vi "EnableDisable RTM.vi"(8 "error in (no error)":errorcluster, 11 "Node Ptr":T1 format="%.0x") -> (0 "error out":errorcluster)   [LabVIEW 2020, in "AIM ARINC 429 System Explorer.lvlib" / "Implementation.lvlib"]
uses:
  Implementation.lvlib
  <vilib>/NI VeriStand/Custom Device API/Custom Device Item Ref.ctl
  Scripting/AIM/AIM ARINC 429 Scripting.lvlib
  <vilib>/NI VeriStand/Custom Device API/Custom Device API.lvlib
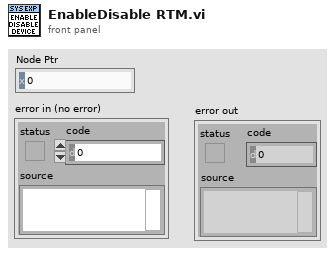
[diagram p1: front panel]
types:
  T1 = typedef "Custom Device API.lvlib/Custom Device Item Ref.ctl" = u64
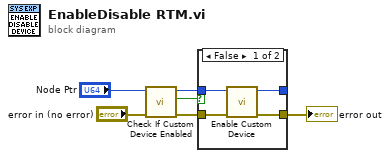
[diagram p0: block diagram]
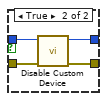
[diagram p2: hidden frame]
diagram:
  n1 = call "Check If Custom Device Enabled.vi"("error in (no error)"="error in (no error)", "AIM ARINC 429 ref"="Node Ptr") -> ("error out"=w2:errorcluster, "Is Custom Device Enabled?"=w4:bool, "AIM ARINC 429 ref"=w3:T1)  [unwired: 7 in]
  n2 = case shown="False" w4 {
    tunnel: w3 -> [w10 w13]
    tunnel: w2 -> [w9 w14]
    tunnel: [w7 w12] -> _
    tunnel: [w8 w11] -> w1
    frame False {
      n3 = call "Enable Custom Device.vi"("error in (no error)"=w9, "AIM ARINC 429 ref"=w10) -> ("error out"=w8:errorcluster, "AIM ARINC 429 ref out"=w7:T1)  [unwired: 8 in]
    }
    frame True {
      n4 = call "Disable Custom Device.vi"("error in (no error)"=w14, "AIM ARINC 429 ref"=w13) -> ("error out"=w11:errorcluster, "AIM ARINC 429 ref out"=w12:T1)  [unwired: 8 in]
    }
  }
  "error out" <- w1
